vi "CheezyAtan.vi"(1 "arg":dbl) -> (0 "atan(arg)":dbl)   [LabVIEW 2015]
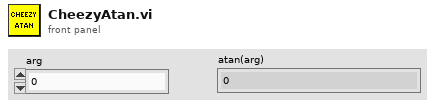
[diagram p1: front panel]
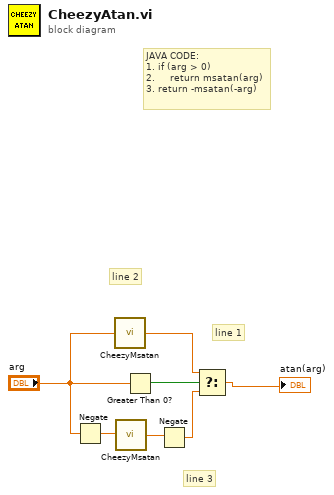
[diagram p0: block diagram]
diagram:
  # "line 3"
  # "line 2"
  # "line 1"
  # "JAVA CODE:\n1. if (arg > 0)\n2.     return msatan(arg)\n3. return -msatan(-arg)"
  n1 = Negate(x="arg") -> (-x=w3:dbl)
  n2 = call <userlib>:"CheezyMsatan.vi"("arg"="arg") -> ("msatan(arg)"=w6:dbl)
  n3 = call <userlib>:"CheezyMsatan.vi"("arg"=w3) -> ("msatan(arg)"=w5:dbl)
  n4 = Greater Than 0?(x="arg") -> (x > 0?=w7:bool)
  n5 = Negate(x=w5) -> (-x=w4:dbl)
  n6 = Select(t=w6, s=w7, f=w4) -> (s? t:f=→"atan(arg)":dbl)
